vi "Generator.Staircase.vi"(9 "reset?":bool, 10 "period":dbl=10.0 format="%#_13g", 11 "dimension size":i32=1000) -> (3 "Array":dbl[](array[numeric]))   [LabVIEW 2019, in "Generator.lvclass"]
uses:
  <vilib>/Analysis/1siggen.llb/Ramp Pattern by Samples.vi
  Generator.lvclass
  <vilib>/Analysis/NI_AALBase.lvlib
panel:
  out "Waveform Graph":dbl[](graph)
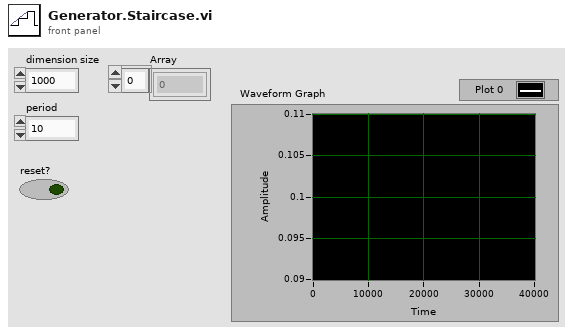
[diagram p1: front panel]
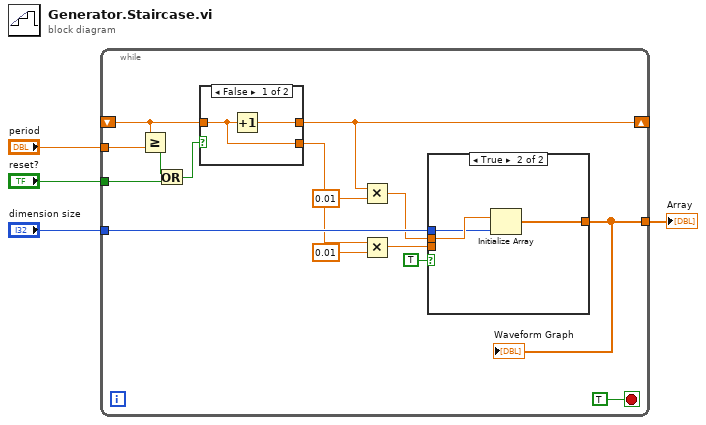
[diagram p0: block diagram]
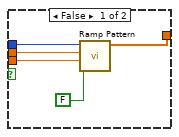
[diagram p2: hidden frame]
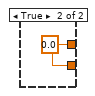
[diagram p3: hidden frame]
diagram:
  n1 = while {
    shift-right: [w9] -> _
    shift-left: _ -> [w17]
    tunnel: [w5] -> w4
    tunnel: "dimension size" -> [w16]
    tunnel: "period" -> [w15]
    tunnel: "reset?" -> [w14]
    stop <- TRUE stop-if-true
    n2 = Greater Or Equal?(x=w17, y=w15) -> (x >= y?=w13:bool)
    n3 = Or(x=w13, y=w14) -> (x .or. y?=w12:bool)
    n4 = case shown="False" w12 {
      tunnel: [w29 w30] -> w9
      tunnel: w17 -> [w28 _]
      tunnel: [w28 w30] -> w7
      frame False {
        n5 = Increment(x=w28) -> (x+1=w29:dbl)
      }
      frame True {
        w30 = 0.0
      }
    }
    n6 = Multiply(x=w9, y=0.01 ("x")) -> (x*y=w10:dbl)
    n7 = Multiply(x=w7, y=0.01 ("x")) -> (x*y=w6:dbl)
    n8 = case shown="True" TRUE {
      tunnel: w10 -> [w22 w27]
      tunnel: [w24 w26] -> w5
      tunnel: w16 -> [w23 w25]
      tunnel: w6 -> [w21 _]
      frame False {
        n9 = call-poly <vilib>:"Ramp Pattern.vi"("exclude end?"=FALSE, "start"=w21, "end"=w22, "samples"=w23) -> ("Ramp Pattern"=w24:dbl[])  [unwired: 6 in, 1 out]
      }
      frame True {
        n10 = Initialize Array(w27, w25) -> (w26:dbl[])
      }
    }
    "Waveform Graph" <- w5
  }
  "Array" <- w4
